vi "Init.vi"(7 "I2C #":T1=-1, 8 "error in (no error)":errorcluster, 10 "Session In":refnum<class "Session.lvclass">) -> (0 "error out":errorcluster, 2 "2D Picture":picture, 3 "64x128 I2C OLED SSD1315 Out":refnum<class "64x128 I2C OLED SSD1315.lvclass">)   [LabVIEW 2020, in "CTI-Peripheral.lvlib" / "64x128 I2C OLED SSD1315.lvclass"]
uses:
  64x128 I2C OLED SSD1315.lvclass
  CTI/Session/Session.lvclass
  CTI/I2C Number.ctl
  CTI/I2C Address.ctl
  Data Types/OLED Size.ctl
  CTI/I2C Connection/I2C Connection.lvclass/I2C Connection.ctl
  64x128 I2C OLED SSD1315.lvclass/64x128 I2C OLED SSD1315.ctl
  CTI/I2C Connection/I2C Connection.lvclass
  CTI/CTI.lvlib
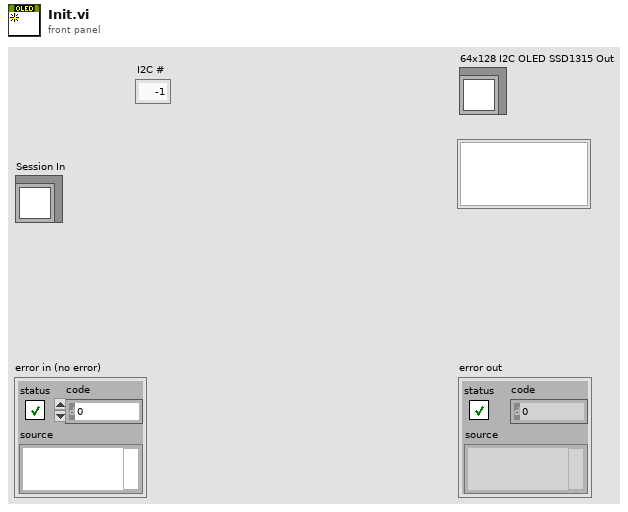
[diagram p1: front panel]
types:
  T1 = typedef "CTI.lvlib/I2C Number.ctl" = i8
  T2 = typedef "CTI-Peripheral.lvlib/64x128 I2C OLED SSD1315.lvclass/OLED Size.ctl" = cluster{"Rows":u8, "Cols":u8}
  T3 = typedef "CTI.lvlib/I2C Address.ctl" = u8
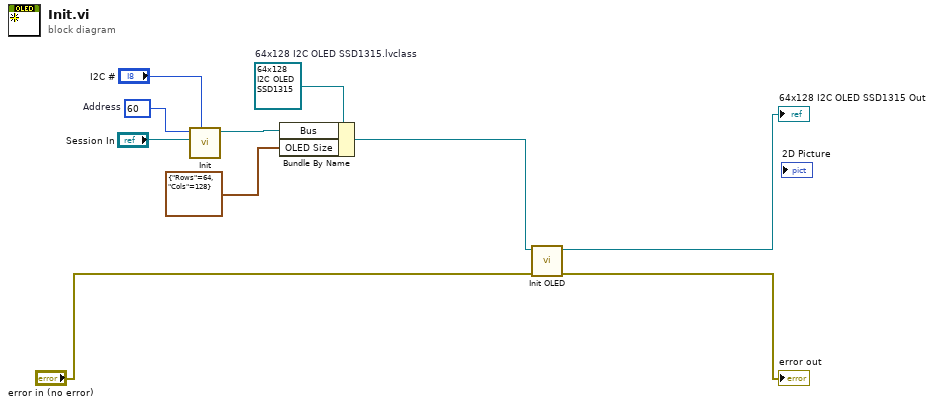
[diagram p0: block diagram]
diagram:
  w6 = refnum<class "64x128 I2C OLED SSD1315.lvclass"> refnum  # 64x128 I2C OLED SSD1315.lvclass
  w7 = T3 60  # Address
  n1 = call "Init.vi"("I2C #"="I2C #", "Session"="Session In", "Address"=w7) -> ("I2C Connection"=w10:refnum<class "I2C Connection.lvclass">)  [unwired: 7 in, 1 out]
  n2 = Bundle By Name(cluster=w6, "Bus"=w10, "OLED Size"=T2 {"Rows"=64, "Cols"=128}) -> (w4:refnum<class "64x128 I2C OLED SSD1315.lvclass">)
  n3 = call "Init OLED.vi"("error in (no error)"="error in (no error)", "64x128 I2C OLED SSD1315 in"=w4) -> ("error out"=→"error out":errorcluster, "64x128 I2C OLED SSD1315 out"=→"64x128 I2C OLED SSD1315 Out":refnum<class "64x128 I2C OLED SSD1315.lvclass">)  [unwired: 7 in, 1 out]
